vi "Close.vi"(8 "error in (no error)":errorcluster, 11 "Bronkhorst Settings in":T1) -> (0 "error out":errorcluster, 3 "Bronkhorst Settings out":T1)   [LabVIEW 2018]
uses:
  Bronkhorst M13 Flow Meter/Settings Cluster.ctl
  Bronkhorst M13 Flow Meter/Bronkhorst M13 Flow Meter.lvlib
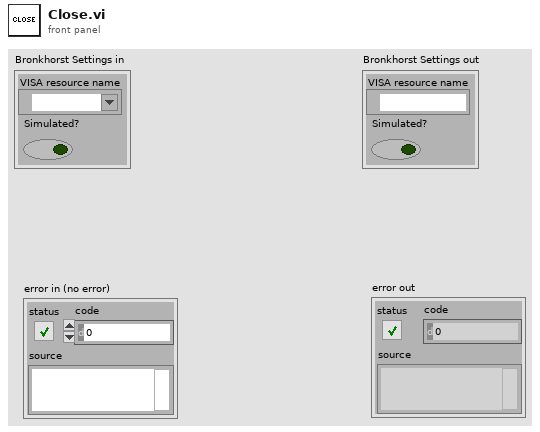
[diagram p1: front panel]
types:
  T1 = typedef "Bronkhorst M13 Flow Meter.lvlib/Settings Cluster.ctl" = cluster{"VISA resource name":refnum<visa-resource-name>, "Simulated?":bool}
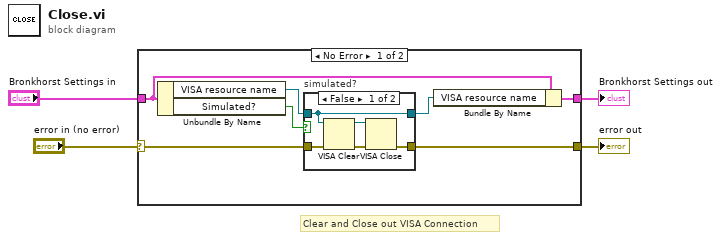
[diagram p0: block diagram]
diagram:
  # "Clear and Close out VISA Connection"
  n1 = case shown="No Error" "error in (no error)" {
    selector: "error in (no error)" -> [w10 w20]
    tunnel: [w9 w20] -> w4
    tunnel: [w8 w19] -> w1
    tunnel: "Bronkhorst Settings in" -> [w7 w19]
    frame No Error {
      n2 = Unbundle By Name(w7) -> ("VISA resource name"=w5:refnum<visa-resource-name>, "Simulated?"=w11:bool)
      n3 = case "simulated?" shown="False" w11 {
        tunnel: [w16 w18] -> w9
        tunnel: w10 -> [w13 w18]
        tunnel: [w15 w17] -> w6
        tunnel: w5 -> [w15 w17]
        frame False {
          n4 = VISA Clear(VISA resource name=w15, error in (no error)=w13) -> (VISA resource name out=w14:refnum<visa-resource-name>, error out=w12:errorcluster)
          n5 = VISA Close(VISA resource name=w14, error in (no error)=w12) -> (error out=w16:errorcluster)
        }
        frame True {
        }
      }
      n6 = Bundle By Name(cluster=w7, "VISA resource name"=w6) -> (w8:T1)
    }
    frame Error {
    }
  }
  "error out" <- w4
  "Bronkhorst Settings out" <- w1
